vi "get_voltages.vi"(8 "error in (no error)":errorcluster, 11 "ImagingModeDL090130Frame in":refnum<class "ImagingModeDL090130Frame.lvclass">) -> (0 "error out":errorcluster, 1 "Vmax_y":dbl, 2 "Vmin_y":dbl, 3 "ImagingModeDL090130Frame out":refnum<class "ImagingModeDL090130Frame.lvclass">, 4 "Vmax_z":dbl, 6 "Vmin_z":dbl)   [LabVIEW 2010, in "ImagingModeDL090130Frame.lvclass"]
uses:
  ImagingModeDL090130Frame.lvclass
  ImagingModeDL090130Frame.lvclass/ImagingModeDL090130Frame.ctl
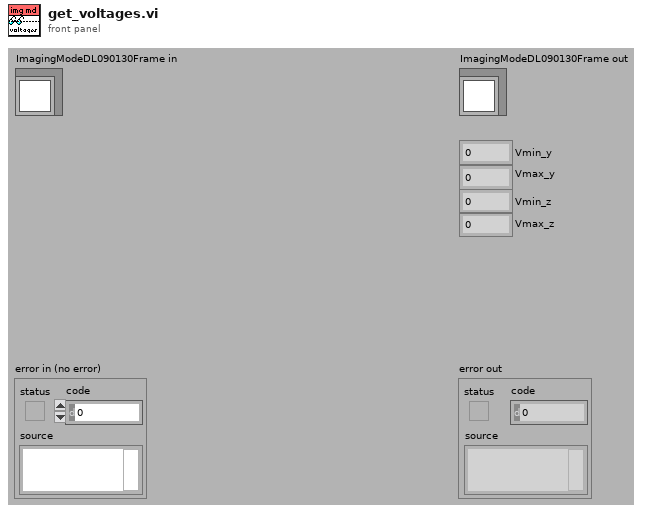
[diagram p1: front panel]
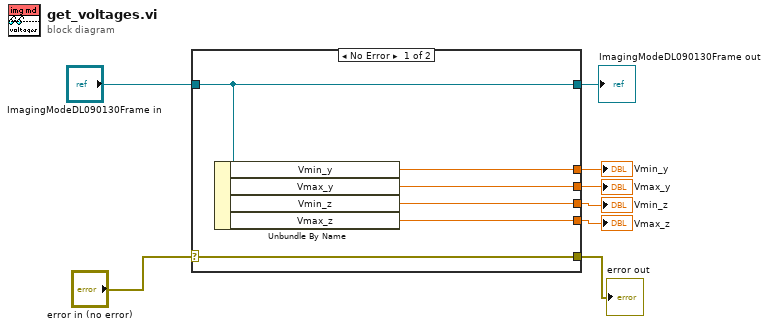
[diagram p0: block diagram]
diagram:
  n1 = case shown="No Error" "error in (no error)" {
    selector: "error in (no error)" -> [w14 w15]
    tunnel: [w14 w15] -> w7
    tunnel: [w13 w16] -> w5
    tunnel: "ImagingModeDL090130Frame in" -> [w13 w16]
    tunnel: [w12 _] -> w4
    tunnel: [w11 _] -> w3
    tunnel: [w10 _] -> w2
    tunnel: [w9 _] -> w1
    frame No Error {
      n2 = Unbundle By Name(w13) -> ("Vmin_y"=w12:dbl, "Vmax_y"=w11:dbl, "Vmin_z"=w10:dbl, "Vmax_z"=w9:dbl)
    }
    frame Error {
    }
  }
  "error out" <- w7
  "ImagingModeDL090130Frame out" <- w5
  "Vmin_y" <- w4
  "Vmax_y" <- w3
  "Vmin_z" <- w2
  "Vmax_z" <- w1
